vi "number to digits (sub vi).vi"(11 "Numeric":dbl) -> (3 "reversed array":dbl[](array[numeric]))   [LabVIEW 2020]
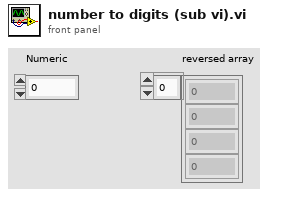
[diagram p1: front panel]
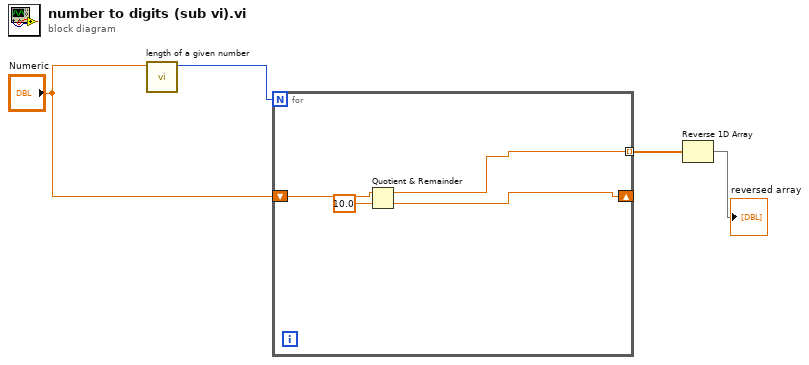
[diagram p0: block diagram]
diagram:
  n1 = call "length of a given number.vi"("Numeric in"="Numeric") -> ("Numeric out"=w1:i32)  [unwired: 10 in]
  n2 = for {
    N: w1 -> [_]
    shift-right: [w6] -> _
    shift-left: "Numeric" -> [w8]
    tunnel: [w5] -> w3 mode=indexing
    n3 = Quotient & Remainder(x=w8, y=10.0) -> (x-y*floor(x/y)=w5:dbl, floor(x/y)=w6:dbl)
  }
  n4 = Reverse 1D Array(array=w3) -> (reversed array=→"reversed array":dbl[])
